vi "Test OpenCVCam.vi"() -> ()   [LabVIEW 2021]
uses:
  OpenCVCam.lvclass
panel:
  in  "Stop":bool
  out "2D Picture":picture
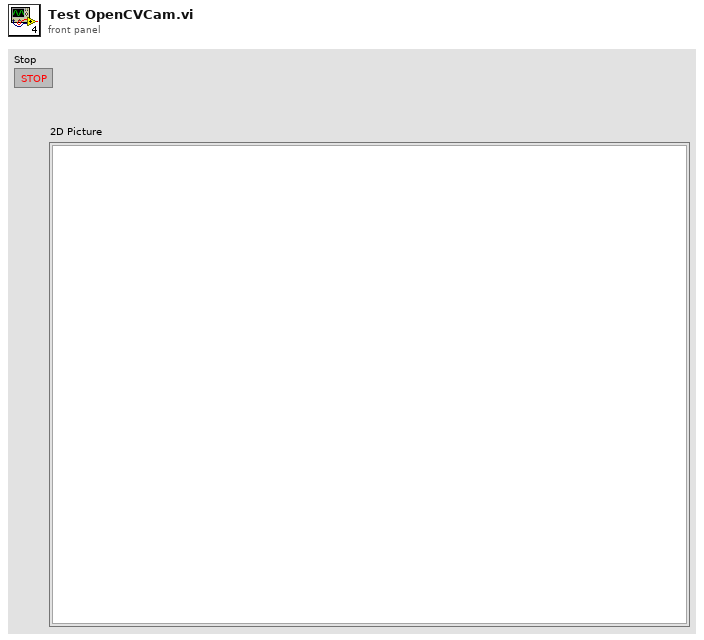
[diagram p1: front panel]
types:
  T1 = typedef "imagedata.ctl" = cluster{"image type":i32, "image depth":i32, "image":u8[], "mask":u8[], "colors":u32[], "Rectangle":cluster{"left":i16, "top":i16, "right":i16, "bottom":i16}}
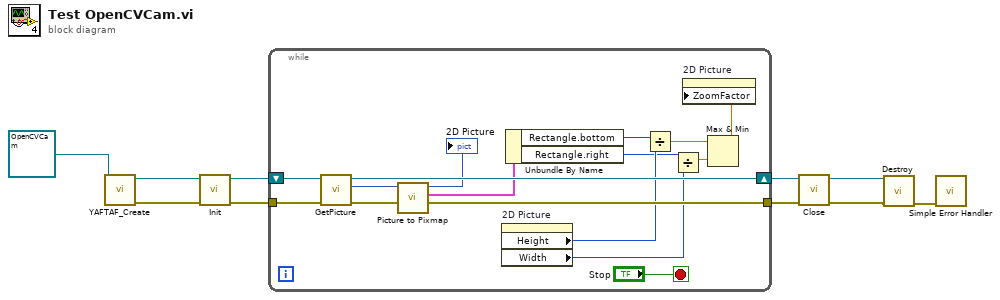
[diagram p0: block diagram]
diagram:
  n1 = call-dynamic "YAFTAF_Create.vi"("ObjectIn"=refnum<class "OpenCVCam.lvclass"> refnum ("OpenCVCam")) -> ("ErrorOut"=w6:errorcluster, "ObjectOut"=w1:refnum<class "OpenCVCam.lvclass">)  [unwired: 9 in]
  n2 = call-dynamic "Init.vi"("ErrorIn"=w6, "OpenCVCamIn"=w1) -> ("ErrorOut"=w10:errorcluster, "OpenCVCamOut"=w5:refnum<class "OpenCVCam.lvclass">)  [unwired: 8 in]
  n3 = while {
    shift-right: [w22] -> w4
    shift-left: w5 -> [w23]
    tunnel: w10 -> [w25]
    tunnel: [w24] -> w9
    stop <- "Stop" stop-if-true
    n4 = call-dynamic "GetPicture.vi"("ErrorIn"=w25, "OpenCVCamIn"=w23) -> ("ErrorOut"=w24:errorcluster, "2D Picture"=w20:picture, "OpenCVCamOut"=w22:refnum<class "OpenCVCam.lvclass">)  [unwired: 7 in]
    n5 = call <vilib>:"Picture to Pixmap.vi"("picture"=w20) -> ("image data"=w18:T1, "new picture"=→"2D Picture":picture)  [unwired: 9 in]
    n6 = property on="2D Picture" class="Pict"() -> ("Height"=w16:u32, "Width"=w14:u32)  [unwired: 2 in, 2 out]
    n7 = Unbundle By Name(w18) -> ("Rectangle.bottom"=w17:i16, "Rectangle.right"=w15:i16)
    n8 = Divide(x=w17, y=w16) -> (x/y=w12:dbl)
    n9 = Divide(x=w15, y=w14) -> (x/y=w13:dbl)
    n10 = Max & Min(x=w12, y=w13) -> (max(x,y)=w11:dbl)  [unwired: 1 out]
    n11 = property on="2D Picture" class="Pict"("ZoomFactor"=w11) -> ()  [unwired: 2 in, 2 out]
  }
  n12 = call-dynamic "Close.vi"("ErrorIn"=w9, "OpenCVCamIn"=w4) -> ("ErrorOut"=w8:errorcluster, "OpenCVCamOut"=w3:refnum<class "OpenCVCam.lvclass">)  [unwired: 8 in]
  n13 = call-dynamic "Destroy.vi"("ErrorIn"=w8, "ObjectIn"=w3) -> ("ErrorOut"=w7:errorcluster)  [unwired: 8 in, 1 out]
  n14 = call <vilib>:"Simple Error Handler.vi"("error in (no error)"=w7) -> ()  [unwired: 4 in, 5 out]
